vi "Main - Update Status (SubVI).vi"(7 "Status":u16(ring) items=["Available", "Running"], 8 "error in":errorcluster, 11 "Machine Name":string) -> (0 "error out":errorcluster)   [LabVIEW 2019]
uses:
  Controls/FGV States.ctl
panel:
  out "data":string[][](array[string])
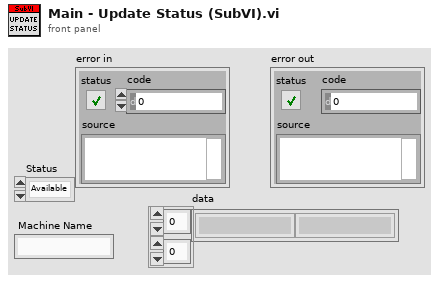
[diagram p1: front panel]
types:
  T1 = typedef "FGV States.ctl" = enum16{"Read", "Write"}
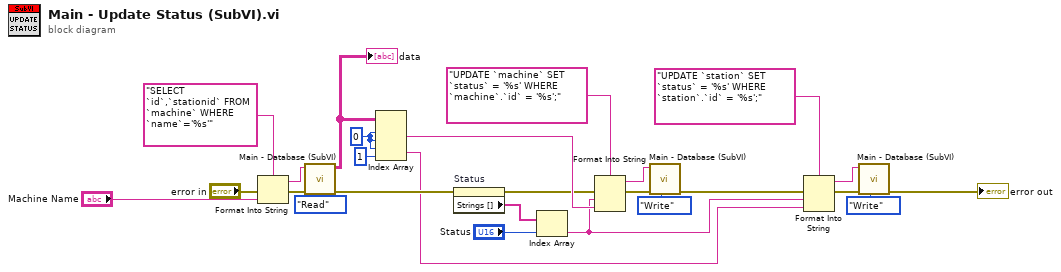
[diagram p0: block diagram]
diagram:
  w17 = 0 ("index (row)")
  n1 = Format Into String(format string="SELECT `id`,`stationid` FROM `machine` WHERE `name`='%s'" ("table"), error in="error in", "Machine Name") -> (resulting string=w21:string, error out=w22:errorcluster)  [unwired: 1 in]
  n2 = call "Main - Database (SubVI).vi"("Enum"=FGV_States."Read", "error in (no error)"=w22, "SQL query"=w21) -> ("error out"=w25:errorcluster, "data"=w23:string[][])  [unwired: 7 in]
  "data" <- w23
  n3 = Index Array(array=w23, index (row) #1=w17, index (col) #1=w17, index (row) #2=w17, index (col) #2=1 ("disabled index (col)")) -> (element #1=w26:string, element #2=w1:string)
  n4 = property on="Status" class="Ring (strict)"(error in=w25) -> (error out=w15:errorcluster, "Strings []"=w13:string[])  [unwired: 1 in, 1 out]
  n5 = Index Array(array=w13, index="Status") -> (element=w2:string)
  n6 = Format Into String(format string="UPDATE `machine` SET `status` = '%s' WHERE `machine`.`id` = '%s';" ("table"), error in=w15, w2, w26) -> (resulting string=w11:string, error out=w12:errorcluster)  [unwired: 1 in]
  n7 = call "Main - Database (SubVI).vi"("Enum"=FGV_States."Write", "error in (no error)"=w12, "SQL query"=w11) -> ("error out"=w5:errorcluster)  [unwired: 7 in, 1 out]
  n8 = Format Into String(format string="UPDATE `station` SET `status` = '%s' WHERE `station`.`id` = '%s';" ("table"), error in=w5, w2, w1) -> (resulting string=w7:string, error out=w6:errorcluster)  [unwired: 1 in]
  n9 = call "Main - Database (SubVI).vi"("Enum"=FGV_States."Write", "error in (no error)"=w6, "SQL query"=w7) -> ("error out"=→"error out":errorcluster)  [unwired: 7 in, 1 out]
